vi "Read_arbitraty_Value.vi"(8 "error in":errorcluster, 10 "Noun(s)":string) -> (0 "error out":errorcluster, 3 "Response":string)   [LabVIEW 2016]
uses:
  Public/Controls/ISOBus Address.ctl
  Instrument_Setup.vi
  Public/Libraries/Temperature/Open/Open Temperature Device.vi
  Global/Global Variables/Data_Display_global.vi
  Mercury iXX.lvlib
  Public/Libraries/Temperature.lvlib
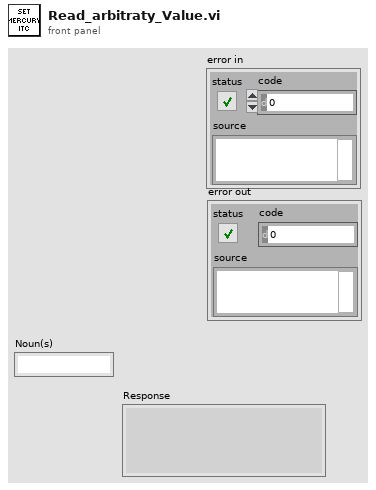
[diagram p1: front panel]
types:
  T1 = typedef "Mercury iXX.lvlib/ISOBus Address.ctl" = i32
  T2 = typedef "Mercury iXX.lvlib/Mercury Reference.ctl" = cluster{"Comms":refnum<visa-resource-name>, "Device ID":string[], "Comms Layer":T3, "Command":string, "Query reference":T4}
  T3 = typedef "Mercury iXX.lvlib/Comms Transport Layer.ctl" = enum16{"Ethernet TCP/IP", "USB", "ISOBus - RS-232", "GPIB"}
  T4 = typedef "Mercury iXX.lvlib/Query Dynamic Reference.ctl" = refnum<vi>
  T5 = typedef "Mercury iXX.lvlib/Response String.ctl" = string
  T6 = typedef "Mercury iXX.lvlib/Is Valid LED.ctl" = bool
  T7 = typedef "20T-VTI-Cluster.ctl" = cluster{"Temperatur (K)":dbl, "Setpoint (K)":dbl, "Rate (K/min)":dbl, "Heater (%)":dbl, "NV (%)":dbl, "Heater Manual":bool, "NV Manual":bool, "Go to Set":bool, "Pressure":dbl, "Dewar Pressure":dbl, "Heater SP":dbl, "D-Heater SP":dbl, "Valid?":bool, "Set Heater SP":bool, "Set NV SP":bool, "Set D-Heater SP":bool, "Dewar Heater Manual":bool, "Heater (%) Display":dbl, "NV (%) Display":dbl, "NV Setpoint":dbl, "Dewar Heater (%)":dbl, "D-Heater (%) Display":dbl, "Change Heater Status":bool, "Change NV Status":bool, "Change D-Heater Status":bool}
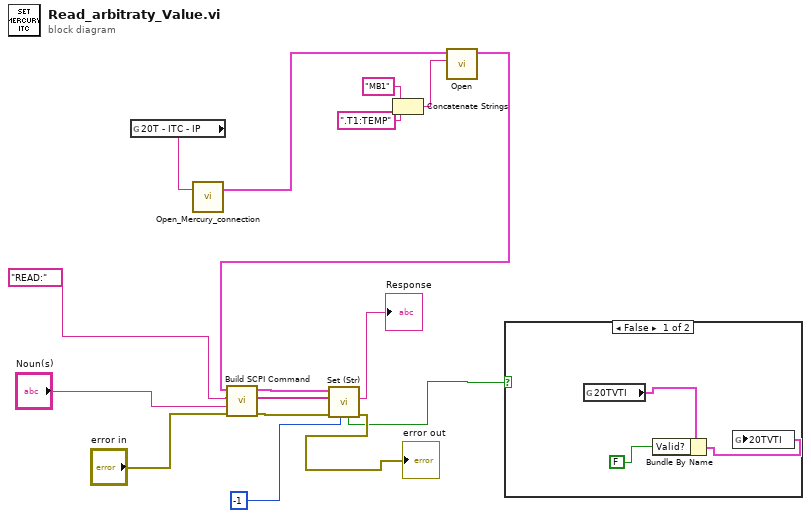
[diagram p0: block diagram]
diagram:
  n1 = global read "Instrument_Setup.vi" "20T - ITC - IP"() -> (w6:string)
  n2 = call "Open_Mercury_connection.vi"("IP Address"=w6) -> ("Mercury Reference Out"=w2:T2)  [unwired: 1 in, 1 out]
  n3 = Concatenate Strings("MB1", ".T1:TEMP" ("Device Identifier")) -> (w3:string)
  n4 = call-poly "Open.vi"("Device Identifier"=w3, "Mercury Reference In"=w2) -> ("Mercury Reference Out"=w1:T2)  [unwired: 2 in, 7 out]
  n5 = call "Build SCPI Command.vi"("error in"="error in", "Noun(s)"="Noun(s)", "Verb"="READ:", "Mercury Reference In"=w1) -> ("error out"=w13:errorcluster, "SCPI Message(s)"=w11:string[], "Mercury Reference Out"=w12:T2)  [unwired: 5 in]
  n6 = call "Set (Str).vi"("ISOBUS address"=T1 -1, "error in"=w13, "SCPI Message(s)"=w11, "Mercury Reference In"=w12) -> ("error out"=→"error out":errorcluster, "Response"=→"Response":T5, "Valid?"=w7:T6)  [unwired: 4 in, 1 out]
  n7 = case shown="False" w7 {
    frame False {
      n8 = global read "Data_Display_global.vi" "20TVTI"() -> (w19:T7)
      n9 = Bundle By Name(cluster=w19, "Valid?"=FALSE) -> (w17:T7)
      n10 = global write "Data_Display_global.vi" "20TVTI"(w17) -> ()
    }
    frame True {
    }
  }
